vi "Configure Setpoint Binary Parameters.vi"(7 "Unit Address (1)":u8=1, 8 "error in (no error)":errorcluster, 9 "Setpoint Value Enabled (False)":bool, 10 "Selected Variable (0: Setpoint Rate Limit Disable)":u8(ring) items=["Setpoint Rate Limit Disable", "Setpoint Tracking Enable", "Alternate Setpoint Enable"], 11 "VISA resource name":refnum<visa-resource-name>) -> (0 "error out":errorcluster, 3 "VISA resource name out":refnum<visa-resource-name>)   [LabVIEW 2014, in "Eurotherm 35xx Series.lvlib"]
doc: "This VI enabled or disabled binary Setpoints Values."
uses:
  <instrlib>/Eurotherm 35xx Series/Eurotherm 35xx Series.lvlib
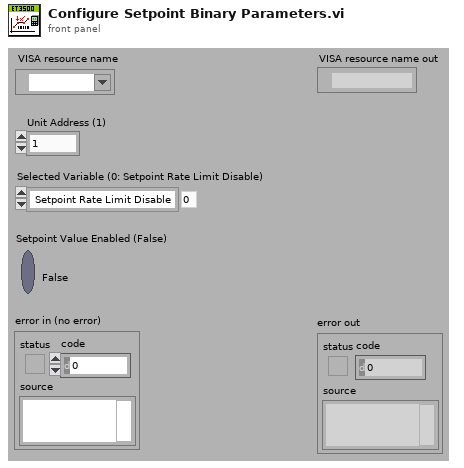
[diagram p1: front panel]
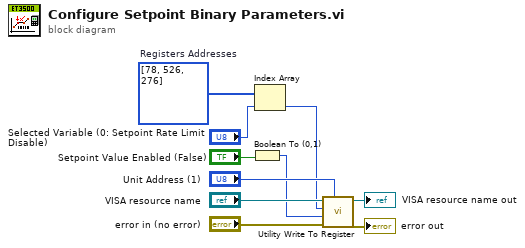
[diagram p0: block diagram]
diagram:
  w3 = u16[] [78, 526, 276]  # Registers Addresses
  n1 = Boolean To (0,1)(Boolean="Setpoint Value Enabled (False)") -> (0, 1=w4:i16)
  n2 = Index Array(array=w3, index="Selected Variable (0: Setpoint Rate Limit Disable)") -> (element=w1:u16)
  n3 = call <instrlib>:"Utility Write To Register.vi"("Unit Address (1)"="Unit Address (1)", "error in (no error)"="error in (no error)", "Data (0)"=w4, "Register Address (0)"=w1, "VISA resource name"="VISA resource name") -> ("error out"=→"error out":errorcluster, "VISA resource name out"=→"VISA resource name out":refnum<visa-resource-name>)  [unwired: 5 in]
